vi "StopSignal-Name.vi"(8 "error in (no error)":errorcluster, 11 "StopSignal":T1) -> (0 "error out":errorcluster, 3 "name":string)   [LabVIEW 2017, in "StopSignal.lvlib"]
uses:
  StopSignal.lvlib
  Typedef/StopSignal.ctl
  Typedef/Action.ctl
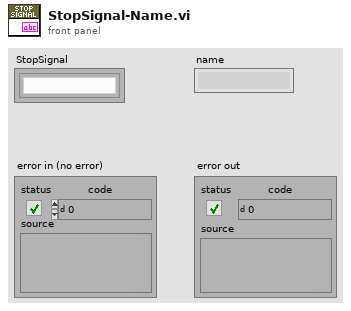
[diagram p1: front panel]
types:
  T1 = typedef "StopSignal.lvlib/StopSignal.ctl" = refnum<k1>
  T2 = typedef "StopSignal.lvlib/Action.ctl" = enum16{"Counter-Increment", "Counter-Decrement", "Counter-Name", "Get-All-Signals-Inorder", "Get-Stop-Signal-Lib"}
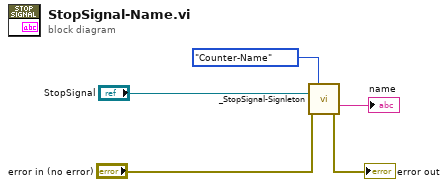
[diagram p0: block diagram]
diagram:
  n1 = call "_StopSignal-Signleton.vi"("Action"=Action."Counter-Name", "StopSignal"="StopSignal", "error in"="error in (no error)") -> ("name"=→"name":string, "error out"=→"error out":errorcluster)  [unwired: 7 in, 4 out]
